vi "Override Pointers.vi"(8 "error in (no error)":errorcluster, 9 "Intermediate Buffer":refnum<class "DBL Pointer.lvclass">, 10 "Inline Buffer":refnum<class "DBL Pointer.lvclass">, 11 "Mock Transfer in":refnum<class "Mock Transfer.lvclass">) -> (0 "error out":errorcluster, 3 "Mock Transfer out":refnum<class "Mock Transfer.lvclass">)   [LabVIEW 2017, in "Mock Transfer.lvclass"]
uses:
  Mock Transfer.lvclass
  C:/github/data-sharing-framework/Data Sharing Framework Core/Engine/Classes/Transfer/Transfer.lvclass
  Engine/Classes/Pointer/DBL Pointer.lvclass
  Engine/Classes/Transfer/Transfer.lvclass/Transfer.ctl
  Engine/Classes/Transfer/Transfer.lvclass
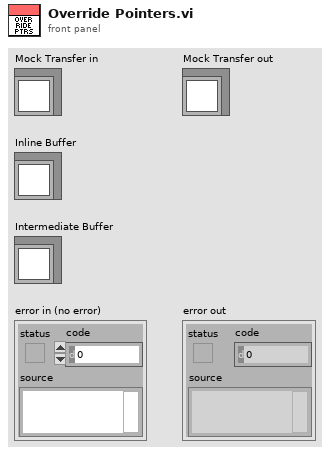
[diagram p1: front panel]
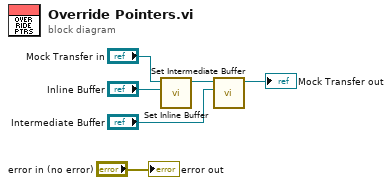
[diagram p0: block diagram]
diagram:
  n1 = call "Set Inline Buffer.vi"("Inline Buffer"="Inline Buffer", "Transfer in"="Mock Transfer in") -> ("Transfer out"=w3:refnum<class "Mock Transfer.lvclass">)  [unwired: 9 in]
  n2 = call "Set Intermediate Buffer.vi"("Intermediate Buffer"="Intermediate Buffer", "Transfer in"=w3) -> ("Transfer out"=→"Mock Transfer out":refnum<class "Mock Transfer.lvclass">)  [unwired: 9 in]
  "error out" <- "error in (no error)"
